vi "CommonVIs RemoveWhiteSpace.vi"(4 "error in (no error)":errorcluster, 5 "Remove from":enum16{"Begining", "End", "Beg+End", "All"}(ring)=enum."All", 6 "Chars to remove":string=" \r\n", 7 "String in":string) -> (0 "error out":errorcluster, 3 "String out":string)   [LabVIEW 2020]
doc: "Remove all specified characters (Chars to remove), found in the input string (String in). The default characters to remove are white spaces (Space, LF, CR).\nThe control \"Remove from\" as 4 options, to specify where in the input string to remove the specified characters.\nBeginning =Removes all specified characters from the beginning of the string, and stops as soon as a none specified characters appears.\nEnd =Starts from the end of the string.\nBeg+End= Removes both from the beginning and end.\nAll= Remove all occurrences of the specified characters inside the string."
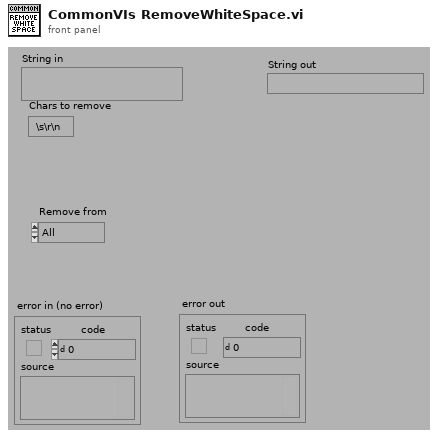
[diagram p1: front panel]
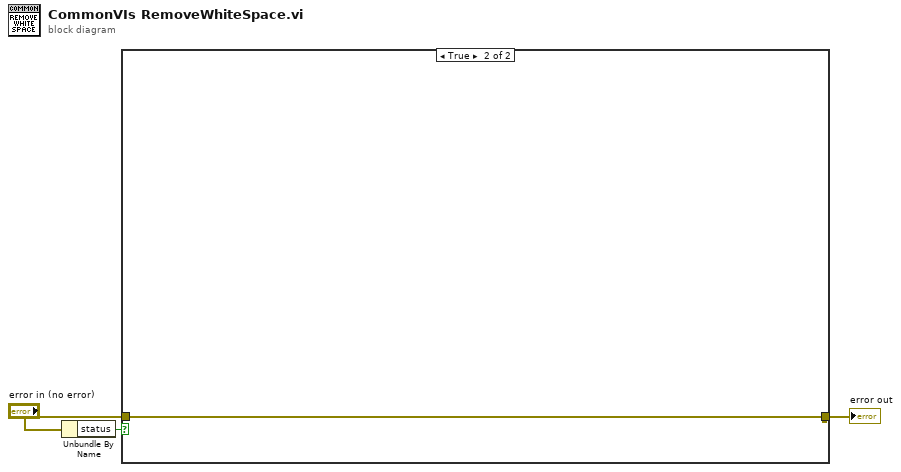
[diagram p0: block diagram]
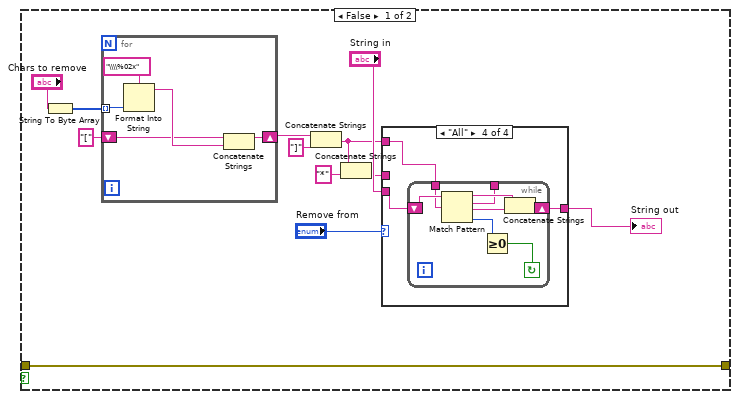
[diagram p2: hidden frame]
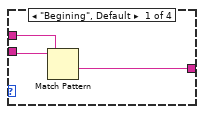
[diagram p3: hidden frame]
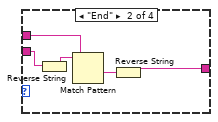
[diagram p4: hidden frame]
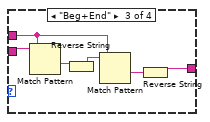
[diagram p5: hidden frame]
diagram:
  n1 = Unbundle By Name("error in (no error)") -> ("status"=w3:bool)
  n2 = case shown="True" w3 {
    tunnel: [w4 w46] -> w2
    tunnel: "error in (no error)" -> [w4 w46]
    frame False {
      n3 = String To Byte Array(string="Chars to remove") -> (unsigned byte array=w13:u8[])
      n4 = for {
        shift-right: [w45] -> w12
        shift-left: "[" -> [w41]
        tunnel: w13 -> [w44] mode=indexing
        n5 = Format Into String(format string="\\\\%02x" ("Format String"), w44) -> (resulting string=w42:string)  [unwired: 2 in, 1 out]
        n6 = Concatenate Strings(w41, w42) -> (w45:string)
      }
      n7 = Concatenate Strings(w12, "]" ("Substring")) -> (w5:string)
      n8 = Concatenate Strings(w5, "*" ("Substring")) -> (w7:string)
      n9 = case shown="\"All\"" "Remove from" {
        tunnel: "String in" -> [w18 w21 w29 w32]
        tunnel: w7 -> [w17 w22 w25 _]
        tunnel: [w16 w19 w24 w31] -> w9
        tunnel: w5 -> [_ _ _ w30]
        frame "Begining", Default {
          n10 = Match Pattern(string=w18, regular expression=w17) -> (after substring=w16:string)  [unwired: 4 out]
        }
        frame "End" {
          n11 = Reverse String(1:w21) -> (0:w23:string)
          n12 = Match Pattern(string=w23, regular expression=w22) -> (after substring=w20:string)  [unwired: 4 out]
          n13 = Reverse String(1:w20) -> (0:w19:string)
        }
        frame "Beg+End" {
          n14 = Match Pattern(string=w29, regular expression=w25) -> (after substring=w26:string)  [unwired: 4 out]
          n15 = Reverse String(1:w26) -> (0:w28:string)
          n16 = Match Pattern(string=w28, regular expression=w25) -> (after substring=w27:string)  [unwired: 4 out]
          n17 = Reverse String(1:w27) -> (0:w24:string)
        }
        frame "All" {
          n18 = while {
            tunnel: [w33] -> _
            tunnel: w30 -> [w39]
            shift-left: w32 -> [w40]
            shift-right: [w36] -> w31
            stop <- w34 continue-if-true
            n19 = Match Pattern(string=w40, regular expression=w39) -> (before substring=w38:string, match substring=w33:string, after substring=w37:string, offset past match=w35:i32)  [unwired: 1 out]
            n20 = Greater Or Equal To 0?(x=w35) -> (x >= 0?=w34:bool)
            n21 = Concatenate Strings(w38, w37) -> (w36:string)
          }
        }
      }
      "String out" <- w9
    }
    frame True {
    }
  }
  "error out" <- w2
